vi "TR to Check.vi"() -> ()   [LabVIEW 2023, in "Network Sync.lvclass"]
uses:
  Network Sync.lvclass
panel:
  in  "Time Reference to Check":string="IEEE 802.1AS-2011_1"
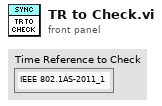
[diagram p1: front panel]
diagram:
